vi "Abort by val.vi"(8 "error in (no error)":errorcluster, 11 "HTTP GET Async.lvclass":refnum<class "GET Async.lvclass">) -> (0 "error out":errorcluster, 3 "HTTP GET Async.lvclass out":refnum<class "GET Async.lvclass">)   [LabVIEW 2019, in "HTTP Client Extensions.lvlib" / "GET Async.lvclass"]
uses:
  GET Async.lvclass
  GET Async.lvclass/GET Async.ctl
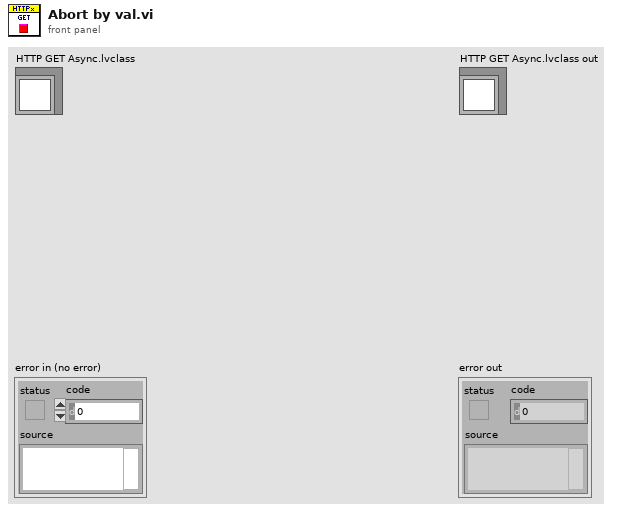
[diagram p1: front panel]
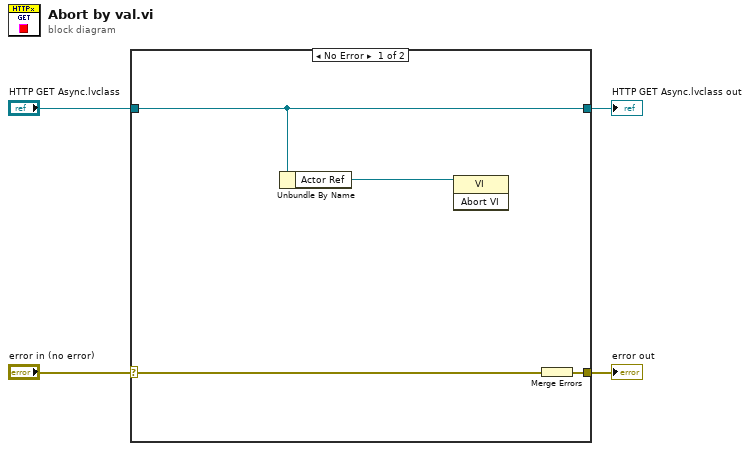
[diagram p0: block diagram]
diagram:
  n1 = case shown="No Error" "error in (no error)" {
    selector: "error in (no error)" -> [w8 w10]
    tunnel: [w7 w10] -> w3
    tunnel: [w5 w9] -> w1
    tunnel: "HTTP GET Async.lvclass" -> [w5 w9]
    frame No Error {
      n2 = Unbundle By Name(w5) -> ("Actor Ref"=w6:refnum<vi>)
      n3 = invoke class="VI" method="Abort VI"(reference=w6) -> ()  [unwired: 2 in, 3 out]
      n4 = Merge Errors(w8) -> (w7:errorcluster)
    }
    frame Error {
    }
  }
  "error out" <- w3
  "HTTP GET Async.lvclass out" <- w1
